vi "epx_Update Vector Data.vi"(8 "error in (no error)":errorcluster, 9 "Display State In":T2={"BGColor"=0, "FGColor"=0, "GridColor"=9868950, "Number of Polar Grids"=12, "Number of Circle Grids"=4, "Vector.Active"=0, "Vectors.Properties"=[], "Height"=0, "Width"=0} {"Number of Circle Grids" min=1 max=100 step=1; "Number of Polar Grids" min=1 max=100 step=1}, 10 "Data In":T1, 11 "Vector Diagram":refnum<vi>) -> (0 "error out":errorcluster, 3 "Vector Diagram out":refnum<vi>)   [LabVIEW 2011, in "NI_EP_Basic.lvlib" / "EPX Vector Diagram.xctl"]
uses:
  <vilib>/addons/Electrical Power/Basic/Controls/Vector Diagram/EPX Vector Diagram.xctl
  <vilib>/addons/Electrical Power/Basic/Controls/Vector Diagram/Abilities/epx_Vector Diagram State.ctl
  <vilib>/addons/Electrical Power/Basic/Controls/Vector Diagram/SubVIs/epx_Vector Type.ctl
  <vilib>/addons/Electrical Power/Basic/Controls/Vector Diagram/Abilities/epx_Vector Diagram Data.ctl
  <vilib>/addons/Electrical Power/Basic/NI_EP_Basic.lvlib
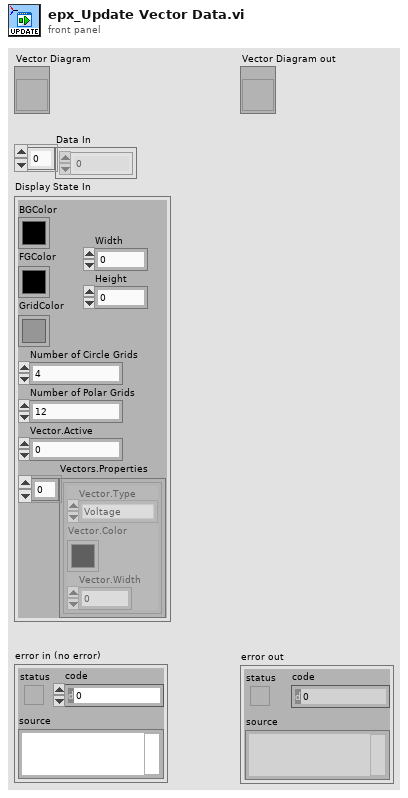
[diagram p1: front panel]
types:
  T1 = typedef "NI_EP_Basic.lvlib/EPX Vector Diagram.xctl/epx_Vector Diagram Data.ctl" = cdb[]
  T2 = typedef "NI_EP_Basic.lvlib/EPX Vector Diagram.xctl/epx_Vector Diagram State.ctl" = cluster{"BGColor":u32, "FGColor":u32, "GridColor":u32, "Number of Polar Grids":i32, "Number of Circle Grids":i32, "Vector.Active":i32, "Vectors.Properties":cluster{"Vector.Type":T3, "Vector.Color":u32, "Vector.Width":u8}[], "Height":u32, "Width":u32}
  T3 = typedef "NI_EP_Basic.lvlib/epx_Vector Type.ctl" = enum16{"Voltage", "Current"}
  T4 = cluster{"BGColor":bool, "FGColor":bool, "GridColor":bool, "Number of Polar Grids":bool, "Number of Circle Grids":bool, "Vector.Active":bool, "Vectors.Properties":cluster{"Vector.Type":bool, "Vector.Color":bool, "Vector.Width":bool}[], "Height":bool, "Width":bool}
  T5 = cluster{"Vector.Type":bool, "Vector.Color":bool, "Vector.Width":bool}[]
  T6 = cluster{"Vector.Type":T3, "Vector.Color":u32, "Vector.Width":u8}[]
  T7 = cluster{"Vector.Type":T3, "Vector.Color":u32, "Vector.Width":u8}
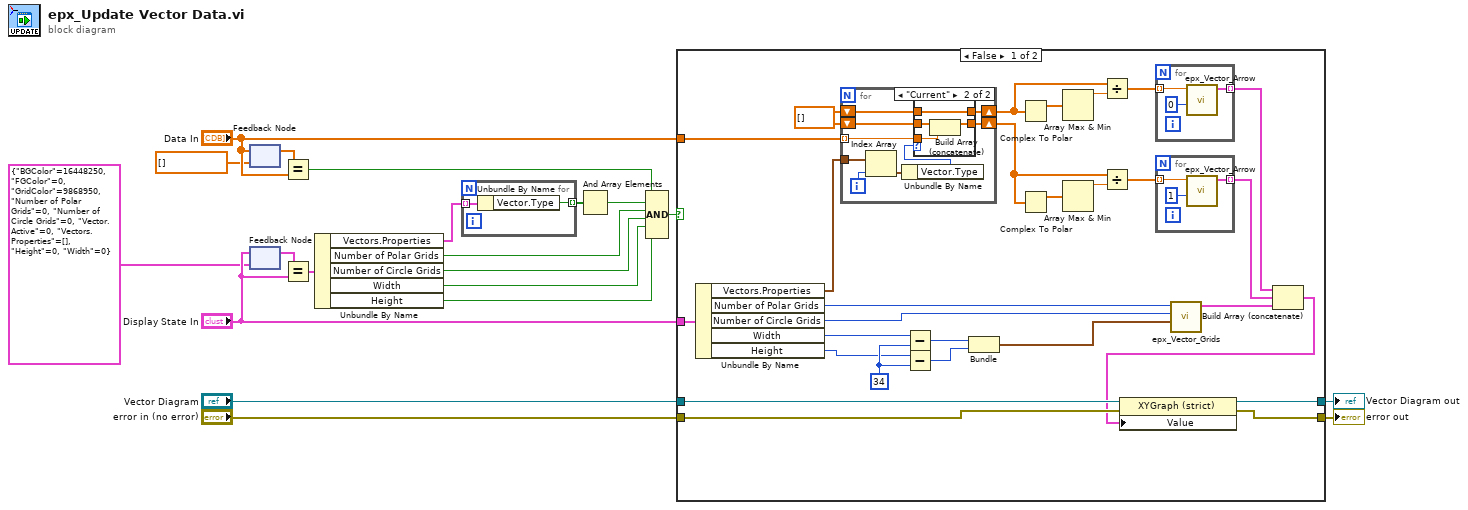
[diagram p0: block diagram]
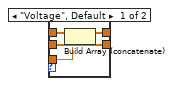
[diagram p2: hidden frame]
diagram:
  n1 = feedback-in #1("Data In") -> ()
  n2 = feedback #1(T1 [] ("Data In")) -> (w16:T1)
  n3 = feedback-in #2("Display State In") -> ()
  n4 = feedback #2(T2 {"BGColor"=16448250, "FGColor"=0, "GridColor"=9868950, "Number of Polar Grids"=0, "Number of Circle Grids"=0, "Vector.Active"=0, "Vectors.Properties"=[], "Height"=0, "Width"=0} ("Display State In")) -> (w14:T2)
  n5 = Equal?(x=w16, y="Data In") -> (x = y?=w11:bool)
  n6 = Equal?(x=w14, y="Display State In") -> (x = y?=w12:T4)
  n7 = Unbundle By Name(w12) -> ("Vectors.Properties"=w10:T5, "Number of Polar Grids"=w7:bool, "Number of Circle Grids"=w6:bool, "Width"=w5:bool, "Height"=w4:bool)
  n8 = for {
    tunnel: w10 -> [w22] mode=indexing
    tunnel: [w21] -> w9 mode=indexing
    n9 = Unbundle By Name(w22) -> ("Vector.Type"=w21:bool)
  }
  n10 = And Array Elements(Boolean array=w9) -> (logical AND=w8:bool)
  n11 = Compound Arithmetic op=AND(w11, w8, w7, w6, w5, w4) -> (w3:bool)
  n12 = case shown="False" w3 {
    tunnel: [w41 w75] -> w20
    tunnel: [w40 w74] -> w19
    tunnel: "Vector Diagram" -> [w38 w74]
    tunnel: "error in (no error)" -> [w37 w75]
    tunnel: "Data In" -> [w30 _]
    tunnel: "Display State In" -> [w32 _]
    frame False {
      w44 = cdb[] []
      w50 = u32 34 ("y")
      n13 = Unbundle By Name(w32) -> ("Vectors.Properties"=w43:T6, "Number of Polar Grids"=w49:i32, "Number of Circle Grids"=w48:i32, "Width"=w36:u32, "Height"=w35:u32)
      n14 = for {
        tunnel: w30 -> [w52] mode=indexing
        tunnel: w43 -> [w59]
        shift-right: [w54] -> w25
        shift-left: w44 -> [w53]
        shift-right: [w56] -> w27
        shift-left: w44 -> [w55]
        i -> [w58]
        n15 = Index Array(array=w59, index=w58) -> (element=w57:T7)
        n16 = Unbundle By Name(w57) -> ("Vector.Type"=w51:T3)
        n17 = case shown="\"Current\"" w51 {
          tunnel: [w63 w64] -> w56
          tunnel: w55 -> [w63 w66]
          tunnel: [w61 w67] -> w54
          tunnel: w53 -> [w62 w67]
          tunnel: w52 -> [w60 w65]
          frame "Voltage", Default {
            n18 = Build Array (concatenate)(w62, w60) -> (w61:cdb[])
          }
          frame "Current" {
            n19 = Build Array (concatenate)(w66, w65) -> (w64:cdb[])
          }
        }
      }
      n20 = Subtract(x=w36, y=w50) -> (x-y=w34:u32)
      n21 = Subtract(x=w35, y=w50) -> (x-y=w33:u32)
      n22 = Bundle(w34, w33) -> (w39:cluster{u32, u32})  [unwired: 1 in]
      n23 = Complex To Polar(r * e^(i*theta)=w25) -> (r=w24:dbl[])  [unwired: 1 out]
      n24 = Complex To Polar(r * e^(i*theta)=w27) -> (r=w46:dbl[])  [unwired: 1 out]
      n25 = Array Max & Min(array=w24) -> (max value=w29:dbl)  [unwired: 3 out]
      n26 = Array Max & Min(array=w46) -> (max value=w28:dbl)  [unwired: 3 out]
      n27 = Divide(x=w25, y=w29) -> (x/y=w23:cdb[])
      n28 = Divide(x=w27, y=w28) -> (x/y=w26:cdb[])
      n29 = for {
        tunnel: w23 -> [w73] mode=indexing
        tunnel: [w72] -> w47 mode=indexing
        n30 = call <vilib>:"epx_Vector_Arrow.vi"("Arrow Type"=u32 0, "Phasor"=w73) -> ("Vector Arow"=w72:cluster{dbl[], dbl[]})  [unwired: 9 in]
      }
      n31 = for {
        tunnel: w26 -> [w70] mode=indexing
        tunnel: [w69] -> w45 mode=indexing
        n32 = call <vilib>:"epx_Vector_Arrow.vi"("Arrow Type"=u32 1, "Phasor"=w70) -> ("Vector Arow"=w69:cluster{dbl[], dbl[]})  [unwired: 9 in]
      }
      n33 = call <vilib>:"epx_Vector_Grids.vi"("Plot Area Size"=w39, "Number of Circle Grids"=w48, "Number of Polar Grids"=w49) -> ("Grids"=w42:cluster{dbl[], dbl[]})  [unwired: 8 in]
      n34 = Build Array (concatenate)(w47, w45, w42) -> (w31:cluster{dbl[], dbl[]}[])
      n35 = property class="XYGraph (strict)"(reference=w38, error in=w37, "Value"=w31) -> (reference out=w40:refnum<vi>, error out=w41:errorcluster)
    }
    frame True {
    }
  }
  "error out" <- w20
  "Vector Diagram out" <- w19
